vi "Get_Comaptibility_Mode.vi"(8 "error in (no error)":errorcluster, 11 "AB_DLL in":refnum<class "AB_DLL.lvclass">) -> (0 "error out":errorcluster, 2 "CompatibilityWith2011":bool, 3 "AB_DLL out":refnum<class "AB_DLL.lvclass">)   [LabVIEW 2020, in "AB_DLL.lvclass"]
uses:
  <vilib>/AppBuilder/AB_Classes/DLL/AB_DLL.lvclass
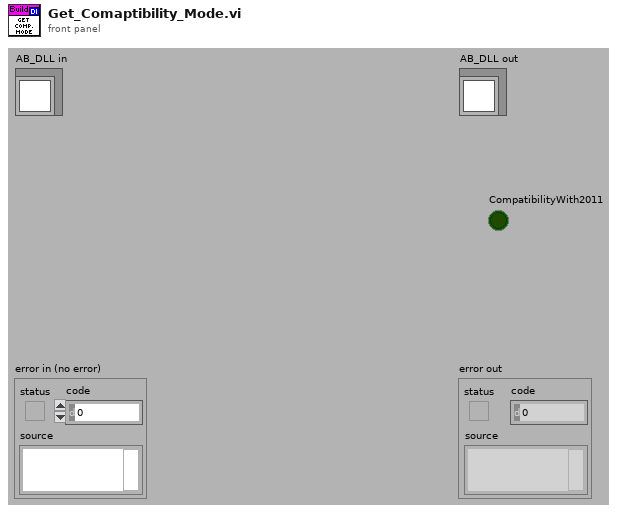
[diagram p1: front panel]
types:
  T1 = typedef "AB_DLL.ctl" = cluster{"delayOSMsg":bool, "includeHeaders":bool, "embeddedRTE":bool, "headerGUID":string, "libGUID":string, "compatibilityWith2011":bool, "includeTypeLibrary":bool, "privateExecutionSystem":bool}
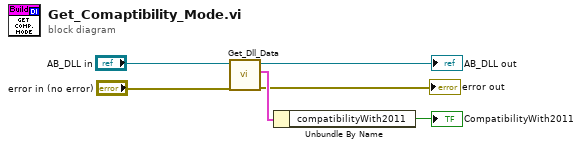
[diagram p0: block diagram]
diagram:
  n1 = call <vilib>:"Get_Dll_Data.vi"("error in (no error)"="error in (no error)", "Class in"="AB_DLL in") -> ("error out"=→"error out":errorcluster, "data"=w5:T1, "Class out"=→"AB_DLL out":refnum<class "AB_DLL.lvclass">)  [unwired: 7 in]
  n2 = Unbundle By Name(w5) -> ("compatibilityWith2011"=→"CompatibilityWith2011":bool)
